vi "Cleanup.vi"(8 "error in (no error)":errorcluster, 11 "Server in":refnum<class "Server.lvclass">) -> (0 "error out":errorcluster)   [LabVIEW 2020, in "HTTP Server.lvlib" / "Server.lvclass"]
uses:
  Server.lvclass
  Server.lvclass/Server.ctl
  Values/Values.lvclass
  Service/Service.lvclass
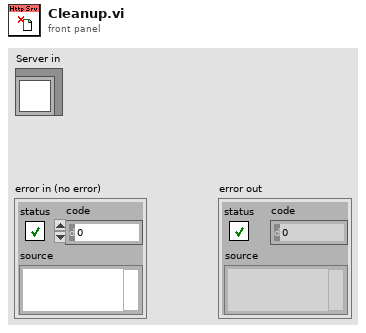
[diagram p1: front panel]
types:
  T1 = typedef "HTTP Server.lvlib/Server.lvclass/Ref Data.ctl" = cluster{"Connection Handler Map":T2, "Request Handler Map":T4, "Route Handler Map":T5, "Controller Handler Map":T6, "Controller Map":T7, "Response Handler Map":T8, "Complete Handler Map":T9, "Exception Handler Map":T10, "Connection Handler Index":u16, "Request Handler Index":u16, "Route Handler Index":u16, "Controller Handler Index":u16, "Controller Index":u16, "Response Handler Index":u16, "Complete Handler Index":u16, "Exception Handler Index":u16, "Values":refnum<class "Values.lvclass">, "Path":path, "Session Type":refnum<class "Session.lvclass">, "Session Cookie Name":string, "WebSocket Handler":refnum<class "WebSocket Handler.lvclass">, "WebSocket Handling":bool, "SSE Handler":refnum<class "SSE Handler.lvclass">, "SSE Handling":bool}
  T2 = typedef "HTTP Server.lvlib/Connection Handler Map.ctl" = map{T3, refnum<class "Connection Handler.lvclass">}
  T3 = typedef "HTTP Server.lvlib/Priority.ctl" = cluster{"Entity":u16, "Index":u16}
  T4 = typedef "HTTP Server.lvlib/Request Handler Map.ctl" = map{T3, refnum<class "Request Handler.lvclass">}
  T5 = typedef "HTTP Server.lvlib/Route Handler Map.ctl" = map{T3, refnum<class "Route Handler.lvclass">}
  T6 = typedef "HTTP Server.lvlib/Controller Handler Map.ctl" = map{T3, refnum<class "Controller Handler.lvclass">}
  T7 = typedef "HTTP Server.lvlib/Controller Map.ctl" = map{T3, refnum<class "Controller.lvclass">}
  T8 = typedef "HTTP Server.lvlib/Response Handler Map.ctl" = map{T3, refnum<class "Response Handler.lvclass">}
  T9 = typedef "HTTP Server.lvlib/Complete Handler Map.ctl" = map{T3, refnum<class "Complete Handler.lvclass">}
  T10 = typedef "HTTP Server.lvlib/Exception Handler Map.ctl" = map{T3, refnum<class "Exception Handler.lvclass">}
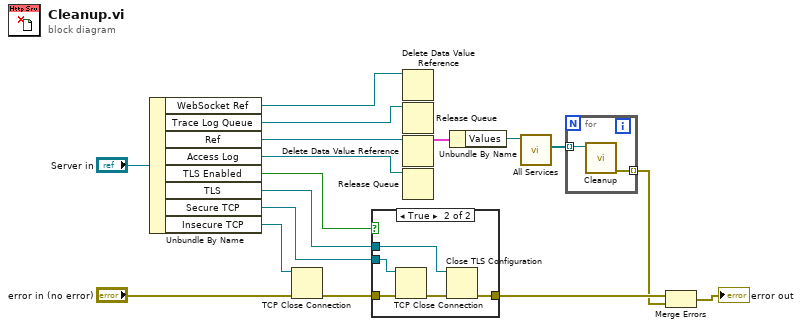
[diagram p0: block diagram]
diagram:
  n1 = Unbundle By Name("Server in") -> ("WebSocket Ref"=w1:refnum<data-value>, "Trace Log Queue"=w2:refnum<queue>, "Ref"=w15:refnum<data-value>, "Access Log"=w16:refnum<queue>, "TLS Enabled"=w3:bool, "TLS"=w4:refnum<k36>, "Secure TCP"=w6:refnum<k5>, "Insecure TCP"=w8:refnum<k5>)
  n2 = TCP Close Connection(connection ID=w8, error in (no error)="error in (no error)") -> (error out=w5:errorcluster)  [unwired: 1 in, 1 out]
  n3 = case shown="True" w3 {
    tunnel: [w18 w19] -> w13
    tunnel: w6 -> [_ w23]
    tunnel: w5 -> [w18 w22]
    tunnel: w4 -> [_ w20]
    frame False {
    }
    frame True {
      n4 = TCP Close Connection(connection ID=w23, error in (no error)=w22) -> (error out=w21:errorcluster)  [unwired: 1 in, 1 out]
      n5 = Close TLS Configuration(8:w21, 11:w20) -> (0:w19:errorcluster)
    }
  }
  n6 = Delete Data Value Reference(data value reference=w1) -> ()  [unwired: 1 in, 2 out]
  n7 = Release Queue(queue=w2) -> ()  [unwired: 2 in, 3 out]
  n8 = Delete Data Value Reference(data value reference=w15) -> (data value=w14:T1)  [unwired: 1 in, 1 out]
  n9 = Release Queue(queue=w16) -> ()  [unwired: 2 in, 3 out]
  n10 = Unbundle By Name(w14) -> ("Values"=w11:refnum<class "Values.lvclass">)
  n11 = call "All Services.vi"("Values in"=w11) -> ("All Services"=w10:refnum<class "Service.lvclass">[])  [unwired: 8 in, 2 out]
  n12 = for {
    tunnel: w10 -> [w25] mode=indexing
    tunnel: [w24] -> w9 mode=indexing
    n13 = call-dynamic "Cleanup.vi"("Service in"=w25) -> ("error out"=w24:errorcluster)  [unwired: 10 in]
  }
  n14 = Merge Errors(w13, w9) -> (→"error out":errorcluster)
